vi "Get Value STR.vi"(0 "Session Handle in":T1, 5 "Lookup String":string, 11 "error in (no error)":errorcluster) -> (4 "Session Handle out":T1, 6 "Value":string, 8 "Exists":bool, 15 "error out":errorcluster)   [LabVIEW 2020, in "HTS.lvlib" / "VariableContainer.lvclass"]
uses:
  VariableContainer.lvclass
  Typedefs/Session Handle.ctl
  VariableContainer.lvclass/VariableContainer.ctl
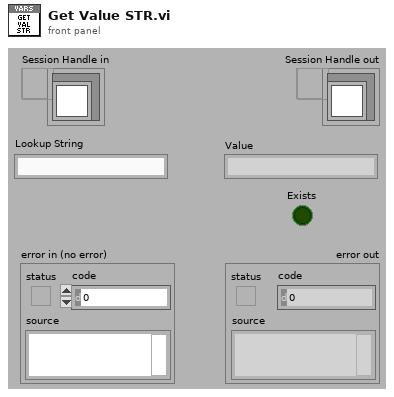
[diagram p1: front panel]
types:
  T1 = typedef "HTS.lvlib/VariableContainer.lvclass/Session Handle.ctl" = refnum<data-value>
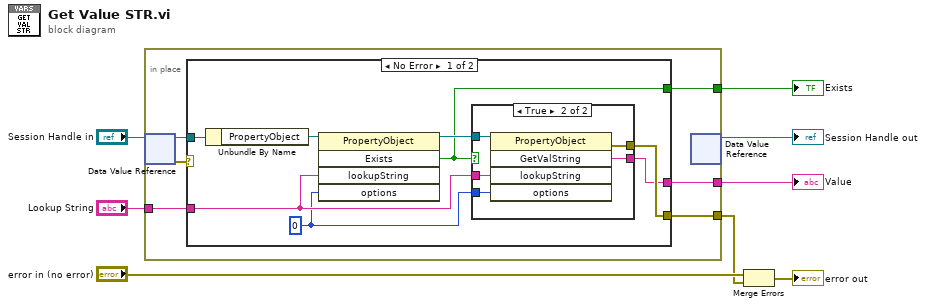
[diagram p0: block diagram]
diagram:
  n1 = in-place {
    in-place-border: "Lookup String" -> [w12]
    in-place-border: [w11] -> w5
    in-place-border: [w10] -> w2
    in-place-border: [w9] -> w1
    n2 = in-place-dvr #1("Session Handle in") -> (w14:refnum<class "VariableContainer.lvclass">, w13:errorcluster)
    n3 = case shown="No Error" w13 {
      selector: w13 -> [_ w28]
      tunnel: w14 -> [w21 _]
      tunnel: w12 -> [w17 _]
      tunnel: [w20 _] -> w11
      tunnel: [w22 w28] -> w10
      tunnel: [w15 _] -> w9
      frame No Error {
        w16 = 0 ("options")
        n4 = Unbundle By Name(w21) -> ("PropertyObject"=w18:refnum<k7>)
        n5 = invoke class="PropertyObject" method="Exists"(reference=w18, "lookupString"=w17, "options"=w16) -> (reference out=w19:refnum<k7>, "Exists"=w15:bool)  [unwired: 2 in, 3 out]
        n6 = case shown="True" w15 {
          tunnel: [_ w27] -> w22
          tunnel: [_ w26] -> w20
          tunnel: w19 -> [_ w25]
          tunnel: w17 -> [_ w24]
          tunnel: w16 -> [_ w23]
          frame False {
          }
          frame True {
            n7 = invoke class="PropertyObject" method="GetValString"(reference=w25, "lookupString"=w24, "options"=w23) -> (error out=w27:errorcluster, "GetValString"=w26:string)  [unwired: 2 in, 3 out]
          }
        }
      }
      frame Error {
      }
    }
    n8 = in-place-dvr #1() -> (→"Session Handle out":T1)  [unwired: 1 in, 1 out]
  }
  "Value" <- w5
  "Exists" <- w1
  n9 = Merge Errors("error in (no error)", w2) -> (→"error out":errorcluster)
